vi "Invert Transformation Matrix.vi"(1 "Transformation Matrix":T1) -> (0 "Inverse of transformation":T1=[[0.2818556107229001, -0.49341675968208987, -0.8228592321708784, 0.11697004227643469], [-0.7778734424176673, -0.6195744782940995, 0.10507318129704712, 0.030499600323496263], [-0.5616674481268332, 0.6104648778688426, -0.5584463363683838, -0.2863453905069739], [0.0, 0.0, 0.0, 1.0]] format="%#_2g")   [LabVIEW 2024]
uses:
  <vilib>/Analysis/Matrix/Datatypes/RealMatrix.ctl
  <vilib>/Analysis/baseanly.llb/A x Vector.vi
  <vilib>/Analysis/baseanly.llb/Real A x B.vi
  <vilib>/Analysis/NI_AALBase.lvlib
  <vilib>/Analysis/Matrix/NI_Matrix.lvlib
panel:
  out "MxM-1":T1=[[0.2818556107229001, -0.49341675968208987, -0.8228592321708784, 0.11697004227643469], [-0.7778734424176673, -0.6195744782940995, 0.10507318129704712, 0.030499600323496263], [-0.5616674481268332, 0.6104648778688426, -0.5584463363683838, -0.2863453905069739], [0.0, 0.0, 0.0, 1.0]] format="%#_2g"
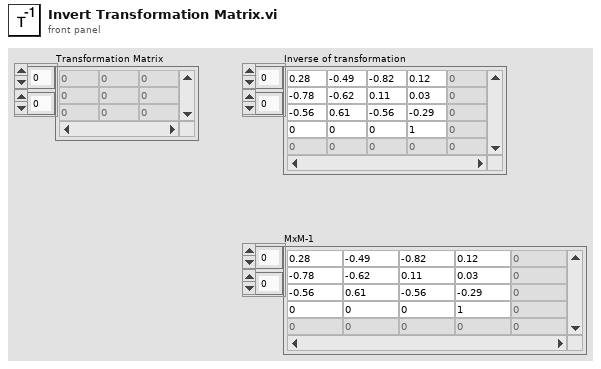
[diagram p1: front panel]
types:
  T1 = typedef "NI_Matrix.lvlib/RealMatrix.ctl" = dbl[][]
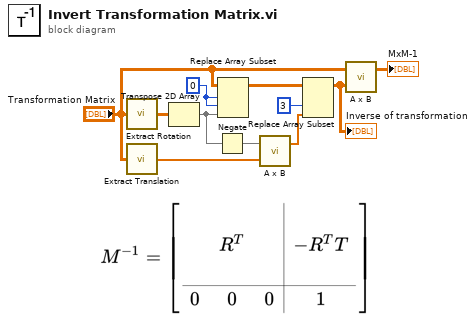
[diagram p0: block diagram]
diagram:
  w10 = 0 ("disabled index (col)")
  n1 = call <userlib>:"Extract Rotation.vi"("Transformation matrix"="Transformation Matrix") -> ("Rotation matrix"=w1:T1)
  n2 = call <userlib>:"Extract Translation.vi"("Transformation matrix"="Transformation Matrix") -> ("Position"=w2:dbl[])
  n3 = Transpose 2D Array(2D array=w1) -> (transposed array=w11:T1)
  n4 = Negate(x=w11) -> (-x=w3:T1)
  n5 = Replace Array Subset(array="Transformation Matrix", new element=w11, index (row)=w10, index (col)=w10) -> (w9:T1)
  n6 = call-poly <vilib>:"A x B.vi"("Vector"=w2, "A"=w3) -> ("A x Vector"=w5:dbl[])  [unwired: 1 out]
  n7 = Replace Array Subset(array=w9, new element=w5, index (col)=3 ("disabled index (col)")) -> (w6:T1)  [unwired: 1 in]
  "Inverse of transformation" <- w6
  n8 = call-poly <vilib>:"A x B.vi"("B"=w6, "A"="Transformation Matrix") -> ("A x B"=→"MxM-1":T1)  [unwired: 1 out]
